vi "Write Communications Configuration.vi"(8 "error in (no error)":errorcluster, 10 "Configuration":T1={"Subscribe to modules"=["Spectrum Recorder", "Line Detector"]}, 11 "Communications in":refnum<class "Communications.lvclass">) -> (0 "error out":errorcluster, 3 "Communications out":refnum<class "Communications.lvclass">)   [LabVIEW 2016, in "Communications.lvclass"]
uses:
  Communications.lvclass
  Communications Configuration.ctl
  Communications.lvclass/Communications.ctl
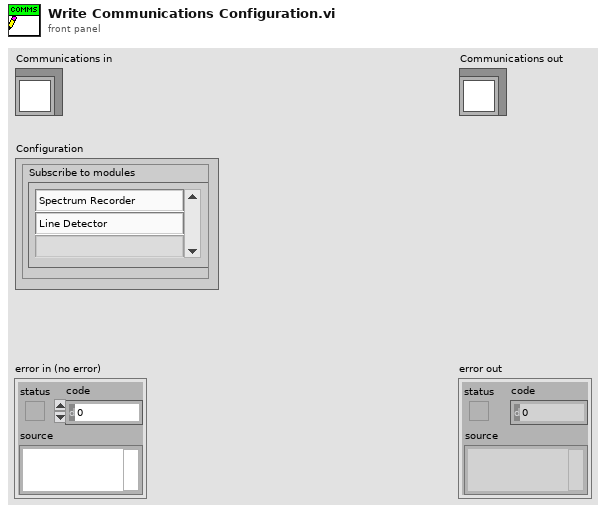
[diagram p1: front panel]
types:
  T1 = typedef "Communications Configuration.ctl" = cluster{"Subscribe to modules":string[]}
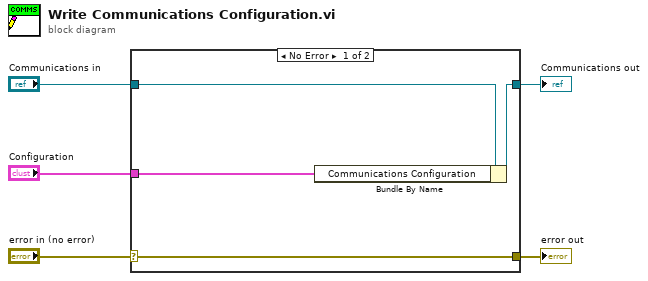
[diagram p0: block diagram]
diagram:
  n1 = case shown="No Error" "error in (no error)" {
    selector: "error in (no error)" -> [w9 w10]
    tunnel: [w9 w10] -> w4
    tunnel: [w7 w11] -> w2
    tunnel: "Communications in" -> [w8 w11]
    tunnel: "Configuration" -> [w6 _]
    frame No Error {
      n2 = Bundle By Name(cluster=w8, "Communications Configuration"=w6) -> (w7:refnum<class "Communications.lvclass">)
    }
    frame Error {
    }
  }
  "error out" <- w4
  "Communications out" <- w2
